vi "RDV-init.vi"(8 "error in (no error)":errorcluster, 11 "RDV-Reflection_Data_viewer in":refnum<class "RDV-Reflection_Data_viewer.lvclass">) -> (0 "error out":errorcluster, 3 "RDV-Reflection_Data_viewer out":refnum<class "RDV-Reflection_Data_viewer.lvclass">)   [LabVIEW 2020, in "RDV-Reflection_Data_viewer.lvclass"]
uses:
  RDV-Reflection_Data_viewer.lvclass
  RDV-Reflection_Data_viewer.lvclass/RDV-Reflection_Data_viewer.ctl
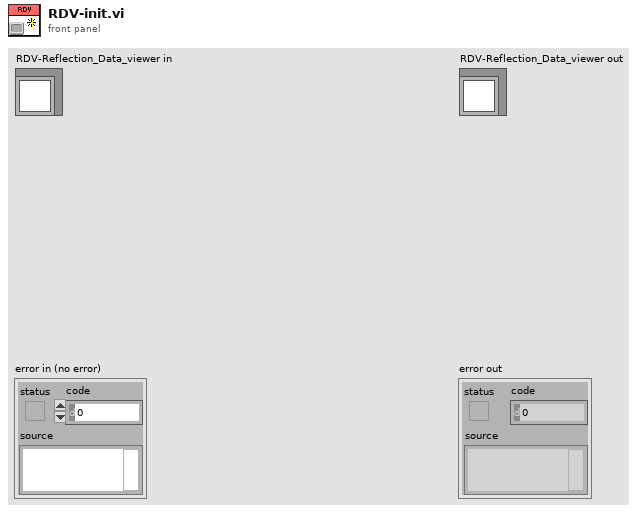
[diagram p1: front panel]
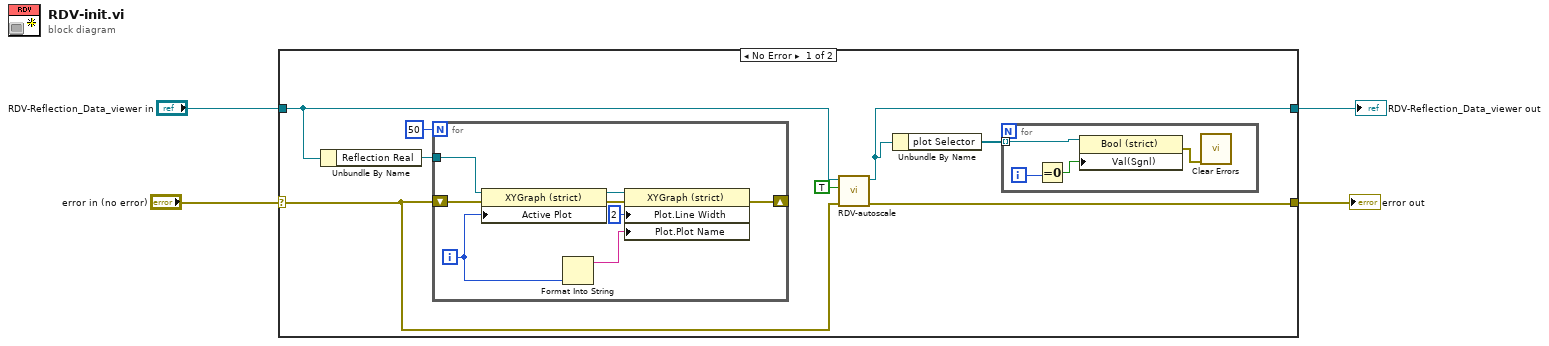
[diagram p0: block diagram]
diagram:
  n1 = case shown="No Error" "error in (no error)" {
    selector: "error in (no error)" -> [w10 w26]
    tunnel: [w9 w26] -> w3
    tunnel: [w6 w25] -> w1
    tunnel: "RDV-Reflection_Data_viewer in" -> [w8 w25]
    frame No Error {
      n2 = Unbundle By Name(w8) -> ("Reflection Real"=w12:refnum<vi>)
      n3 = for {
        N: 50 -> [_]
        tunnel: w12 -> [w20]
        shift-right: [w17] -> _
        shift-left: w10 -> [w19]
        i -> [w21]
        n4 = property on="Property Node" class="XYGraph (strict)"(reference=w20, error in=w19, "Active Plot"=w21) -> (reference out=w23:refnum<vi>, error out=w24:errorcluster)
        n5 = Format Into String(w21) -> (resulting string=w18:string)  [unwired: 3 in, 1 out]
        n6 = property on="Property Node" class="XYGraph (strict)"(reference=w23, error in=w24, "Plot.Line Width"=u8 2, "Plot.Plot Name"=w18) -> (error out=w17:errorcluster)  [unwired: 1 out]
      }
      n7 = call "RDV-autoscale.vi"("error in (no error)"=w10, "Autoscale"=TRUE, "RDV-Reflection_Data_viewer in"=w8) -> ("error out"=w9:errorcluster, "RDV-Reflection_Data_viewer out"=w6:refnum<class "RDV-Reflection_Data_viewer.lvclass">)  [unwired: 7 in]
      n8 = Unbundle By Name(w6) -> ("plot Selector"=w5:refnum<vi>[])
      n9 = for {
        tunnel: w5 -> [w15] mode=indexing
        i -> [w16]
        n10 = Equal To 0?(x=w16) -> (x = 0?=w14:bool)
        n11 = property on="Property Node" class="Bool (strict)"(reference=w15, "Val(Sgnl)"=w14) -> (error out=w13:errorcluster)  [unwired: 1 in, 1 out]
        n12 = call <vilib>:"Clear Errors.vi"("error in (no error)"=w13) -> ()  [unwired: 5 in, 2 out]
      }
    }
    frame Error {
    }
  }
  "error out" <- w3
  "RDV-Reflection_Data_viewer out" <- w1
